vi "From CSV File.vi"(8 "error in (no error)":errorcluster, 9 "Path":path, 10 "engine configuration":refnum<class "engine configuration.lvclass">, 11 "module editor node in":refnum<class "module editor node.lvclass">) -> (0 "error out":errorcluster, 2 "Update":bool, 3 "module editor node out":refnum<class "module editor node.lvclass">)   [LabVIEW 2014, in "PL Framework Configuration Tool.lvlib" / "module editor node.lvclass"]
uses:
  module editor node.lvclass
  <vilib>/NI/Module Execution Interface/Engine Configuration/engine configuration.lvclass
  <vilib>/NI/Tag Bus Module Framework/module configuration/TBM module configuration.lvclass
  <vilib>/NI/Configuration Framework/serializable configuration/NISE_CEF_serializable configuration.lvclass
panel:
  in  "type (empty)":string[][](array[string])
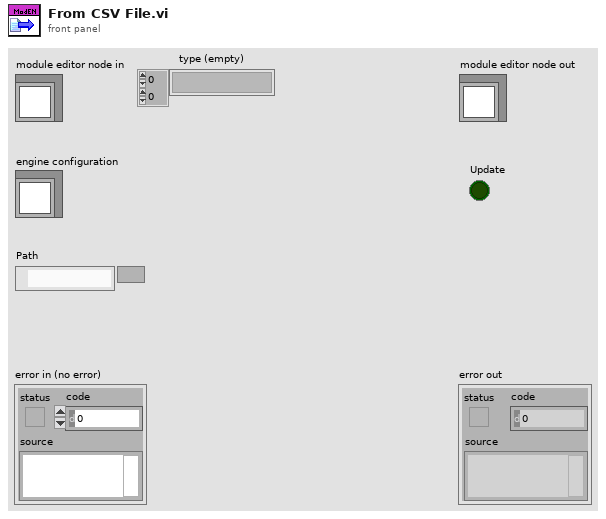
[diagram p1: front panel]
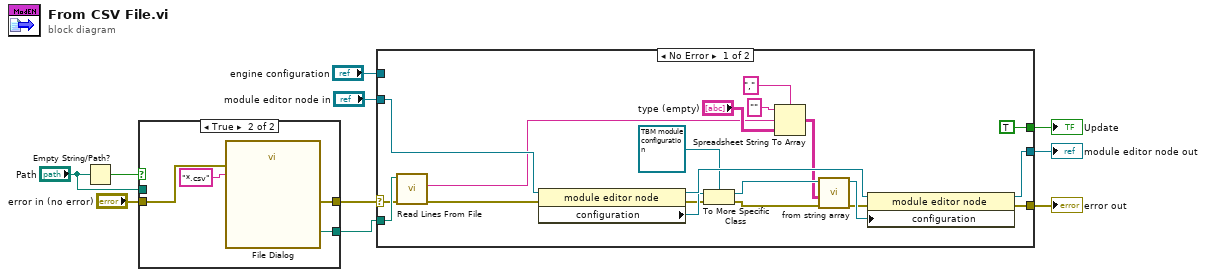
[diagram p0: block diagram]
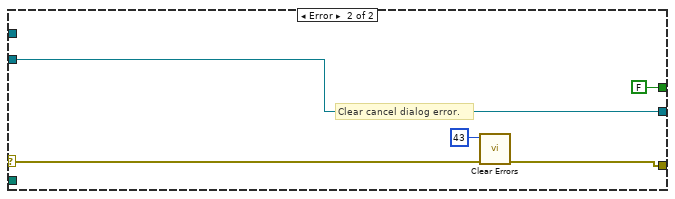
[diagram p3: hidden frame]
diagram:
  n1 = Empty String/Path?(string/path="Path") -> (empty?=w7:bool)
  n2 = case shown="True" w7 {
    tunnel: "error in (no error)" -> [w11 w15]
    tunnel: [w11 w14] -> w5
    tunnel: [w12 w13] -> w4
    tunnel: "Path" -> [w12 _]
    frame False {
    }
    frame True {
      n3 = call "File Dialog"("error in"=w15, "pattern (all files)"="*.csv") -> ("selected path"=w13:path, "error out"=w14:errorcluster)  [unwired: 10 in, 2 out]
    }
  }
  n4 = case shown="No Error" w5 {
    selector: w5 -> [w18 w39]
    tunnel: [w25 w38] -> w10
    tunnel: [w34 w41] -> w8
    tunnel: "module editor node in" -> [w36 w41]
    tunnel: w4 -> [w24 _]
    tunnel: "engine configuration" -> [_ _]
    tunnel: [TRUE ("Update") FALSE ("Update")] -> w2
    frame No Error {
      n5 = call "Read Lines From File.vi"("file path (dialog if empty)"=w24, "error in (not an error)"=w18) -> ("line string"=w22:string, "error out"=w17:errorcluster)  [unwired: 5 in, 1 out]
      n6 = property class="module editor node"(reference=w36, error in=w17) -> (reference out=w35:refnum<class "module editor node.lvclass">, error out=w28:errorcluster, "configuration"=w32:refnum<class "NISE_CEF_serializable configuration.lvclass">)
      n7 = To More Specific Class(target class=refnum<class "TBM module configuration.lvclass"> refnum ("module configuration in"), reference=w32, error in=w28) -> (specific class reference=w31:refnum<class "TBM module configuration.lvclass">, error out=w27:errorcluster)
      n8 = Spreadsheet String To Array(delimiter (Tab)=",", format string="", spreadsheet string=w22, array type (2D Dbl)="type (empty)") -> (array=w19:string[][])
      n9 = call-dynamic "from string array.vi"("error in (no error)"=w27, "String Array"=w19, "module configuration in"=w31) -> ("error out"=w26:errorcluster, "module configuration out"=w30:refnum<class "TBM module configuration.lvclass">)  [unwired: 7 in]
      n10 = property class="module editor node"(reference=w35, error in=w26, "configuration"=w30) -> (reference out=w34:refnum<class "module editor node.lvclass">, error out=w25:errorcluster)
    }
    frame Error {
      # "Clear cancel dialog error."
      n11 = call <vilib>:"Clear Errors.vi"("error in (no error)"=w39, "specific error code to clear (0: all)"=43) -> ("error out"=w38:errorcluster)  [unwired: 4 in, 1 out]
    }
  }
  "error out" <- w10
  "module editor node out" <- w8
  "Update" <- w2
